vi "LimeLite_V2.vi"() -> ()   [LabVIEW 2018]
uses:
  <vilib>/Rock Robotics/Network Tables/NT Read Number.vi
panel:
  out "Total":dbl
  out "Total Area":dbl
  out "Offset Y":dbl
  out "Offset X":dbl
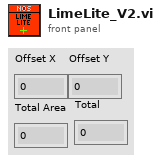
[diagram p1: front panel]
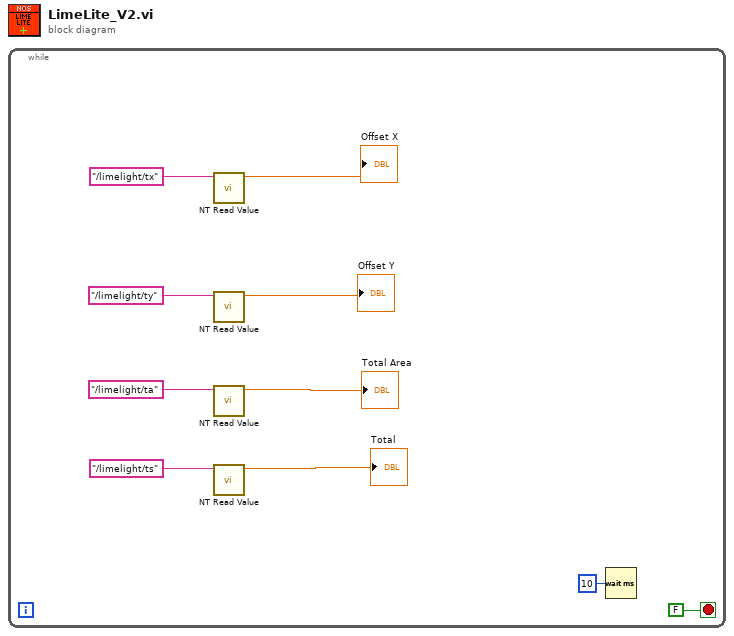
[diagram p0: block diagram]
diagram:
  n1 = while {
    stop <- FALSE stop-if-true
    n2 = call-poly <vilib>:"NT Read Value.vi"("Name"="/limelight/tx") -> ("Numeric"=→"Offset X":dbl)  [unwired: 9 in, 1 out]
    n3 = call-poly <vilib>:"NT Read Value.vi"("Name"="/limelight/ty") -> ("Numeric"=→"Offset Y":dbl)  [unwired: 9 in, 1 out]
    n4 = call-poly <vilib>:"NT Read Value.vi"("Name"="/limelight/ta") -> ("Numeric"=→"Total Area":dbl)  [unwired: 9 in, 1 out]
    n5 = call-poly <vilib>:"NT Read Value.vi"("Name"="/limelight/ts") -> ("Numeric"=→"Total":dbl)  [unwired: 9 in, 1 out]
    n6 = Wait (ms)(milliseconds to wait=u32 10) -> ()  [unwired: 1 out]
  }
